vi "OpenDevice.vi"(8 "error in (no error)":errorcluster, 10 "path":path) -> (0 "error out":errorcluster, 3 "Device Index":u8)   [LabVIEW 2019, in "TopasDriver.lvlib"]
uses:
  TopasDriver.lvlib
  FemtoLabControl/Libraries/Topas/TopasAPI.dll
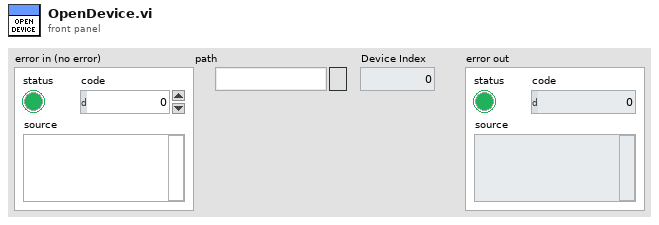
[diagram p1: front panel]
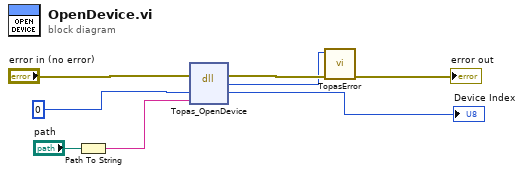
[diagram p0: block diagram]
diagram:
  n1 = Path To String(path="path") -> (string=w3:string)
  n2 = dll-call lib="C:/Users/Michael/Documents/GitHub/CampenLab/FemtoLabControl/Libraries/Topas/TopasAPI.dll" fn="Topas_OpenDevice"(error in="error in (no error)", "index"=u8 0 ("Device Index"), "path"=w3) -> (error out=w6:errorcluster, "return type"=w4:u32, "index"=→"Device Index":u8)  [unwired: 3 in, 1 out]
  n3 = call "TopasError.vi"("error in"=w6, "Error Code"=w4) -> ("error out"=→"error out":errorcluster)  [unwired: 9 in]
